vi "Get Process Variable.vi"(11 "ILC Actuator Cylinder in":refnum<class "ILC Actuator Cylinder.lvclass">) -> (2 "Process Variable":dbl[unit], 3 "ILC Actuator Cylinder out":refnum<class "ILC Actuator Cylinder.lvclass">)   [LabVIEW 2015, in "ILC Actuator Cylinder.lvclass"]
uses:
  ILC Actuator Cylinder.lvclass
  ILC Actuator Cylinder.lvclass/ILC Actuator Cylinder.ctl
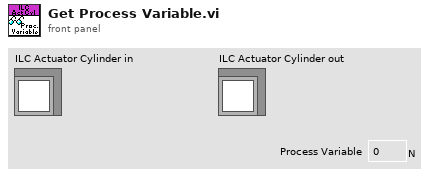
[diagram p1: front panel]
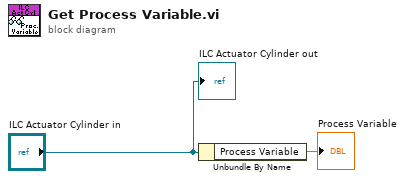
[diagram p0: block diagram]
diagram:
  n1 = Unbundle By Name("ILC Actuator Cylinder in") -> ("Process Variable"=→"Process Variable":dbl[unit])
  "ILC Actuator Cylinder out" <- "ILC Actuator Cylinder in"
